vi "Create Timing Source.vi"   [LabVIEW 2020]
doc: "Creates a 1 kHz, 1MHz, or software-triggered timing source you can use to control the execution of a timed structure. Each timing source has its own unit of timing and/or start time and does not start until the first timed structure that uses the timing source starts. You must manually select the polymorphic instance you want to use."
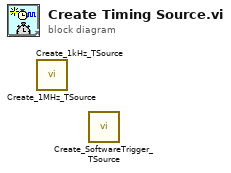
[diagram p0: block diagram]
diagram:
  n1 = call <vilib>:"Create_1MHz_TSource.vi"() -> ()  [unwired: 10 in, 2 out]
  n2 = call <vilib>:"Create_1kHz_TSource.vi"() -> ()  [unwired: 10 in, 2 out]
  n3 = call <vilib>:"Create_SoftwareTrigger_TSource.vi"() -> ()  [unwired: 10 in, 2 out]
